vi "Configure Mask Scaling.vi"(5 "0 Level (0.63 V)":dbl=0.63, 6 "Delta X (118E-9 s)":dbl=1.18e-07 format="%^#_6g", 7 "1 Level (3 V)":dbl=3.0, 8 "error in (no error)":errorcluster, 9 "Initial X (0 s)":dbl, 10 "Enable Bind 1/-1 & 0 Level (T: Enable)":bool=TRUE, 11 "VISA resource name":refnum<visa-resource-name>) -> (0 "error out":errorcluster, 3 "VISA resource name out":refnum<visa-resource-name>)   [LabVIEW 2020, in "Agilent 90000 Series.lvlib"]
doc: "Configures the mask scaling parameters.\n\n<b>Note: </b>\n\nMask testing must be enabled for this VI to operate or a \"Settings Conflict\" error might be thrown. This can be done through the \"Configure Mask Test\" VI."
uses:
  Agilent 90000 Series.lvlib
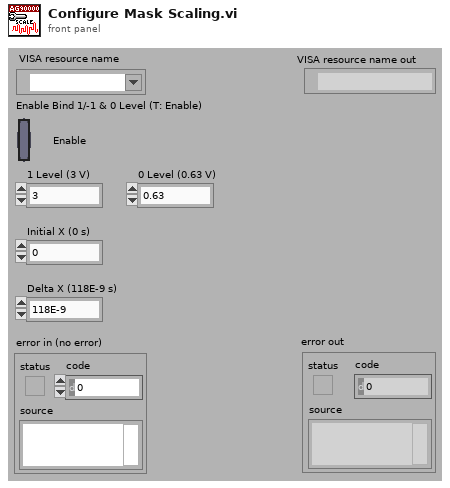
[diagram p1: front panel]
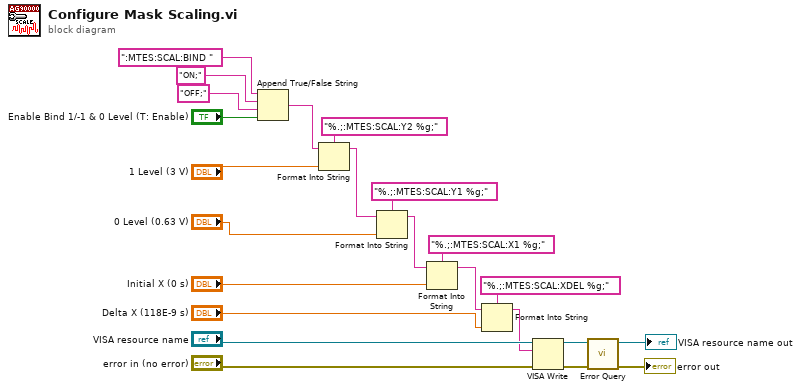
[diagram p0: block diagram]
diagram:
  n1 = Append True/False String(1:"Enable Bind 1/-1 & 0 Level (T: Enable)", 2:"OFF;" ("false string"), 3:"ON;" ("true string"), 4:":MTES:SCAL:BIND " ("string (\"\")")) -> (0:w12:string)
  n2 = Format Into String(format string="%.;:MTES:SCAL:Y2 %g;", initial string=w12, "1 Level (3 V)") -> (resulting string=w2:string)  [unwired: 1 in, 1 out]
  n3 = Format Into String(format string="%.;:MTES:SCAL:Y1 %g;", initial string=w2, "0 Level (0.63 V)") -> (resulting string=w3:string)  [unwired: 1 in, 1 out]
  n4 = Format Into String(format string="%.;:MTES:SCAL:X1 %g;", initial string=w3, "Initial X (0 s)") -> (resulting string=w4:string)  [unwired: 1 in, 1 out]
  n5 = Format Into String(format string="%.;:MTES:SCAL:XDEL %g;", initial string=w4, "Delta X (118E-9 s)") -> (resulting string=w1:string)  [unwired: 1 in, 1 out]
  n6 = VISA Write(VISA resource name="VISA resource name", write buffer=w1, error in (no error)="error in (no error)") -> (VISA resource name out=w21:refnum<visa-resource-name>, error out=w20:errorcluster)  [unwired: 1 out]
  n7 = call "Error Query.vi"("error in (no error)"=w20, "VISA resource name"=w21) -> ("error out"=→"error out":errorcluster, "VISA resource name out"=→"VISA resource name out":refnum<visa-resource-name>)  [unwired: 8 out]
